vi "SetExit.vi"(6 "Legacy (f)?":bool, 8 "error in (no error)":errorcluster) -> (0 "error out":errorcluster)   [LabVIEW 2011]
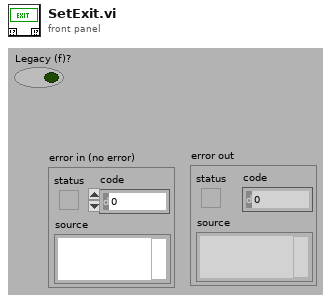
[diagram p1: front panel]
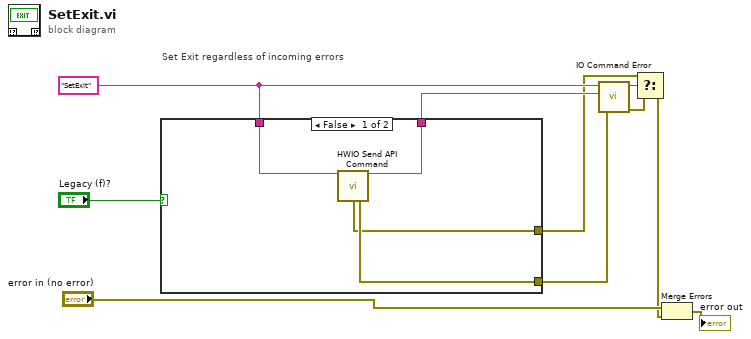
[diagram p0: block diagram]
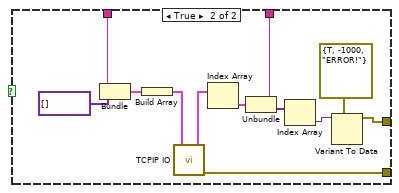
[diagram p2: hidden frame]
diagram:
  w10 = "SetExit"
  # "Set Exit regardless of incoming errors"
  n1 = case shown="False" "Legacy (f)?" {
    tunnel: w10 -> [w12 w24]
    tunnel: [w13 w22] -> w9
    tunnel: [w14 w16] -> w3
    tunnel: [w11 w15] -> w2
    frame False {
      n2 = call "HWIO Send API Command.vi"("Action"=w12) -> ("Action out"=w13:string, "HWError"=w11:errorcluster, "error out"=w14:errorcluster)  [unwired: 7 in, 5 out]
    }
    frame True {
      n3 = Bundle(w24, variant[] []) -> (w25:cluster{string, variant[]})  [unwired: 1 out]
      n4 = Build Array(w25) -> (w20:cluster{string, variant[]}[])
      n5 = call "TCPIP IO.vi"("Commands"=w20) -> ("error out"=w16:errorcluster, "Responses"=w21:cluster{string, variant[]}[])  [unwired: 2 in, 3 out]
      n6 = Index Array(array=w21) -> (element=w23:cluster{string, variant[]})  [unwired: 1 in]
      n7 = Unbundle(w23) -> (w22:string, w17:variant[])
      n8 = Index Array(array=w17) -> (element=w19:variant)  [unwired: 1 in]
      n9 = Variant To Data(type=errorcluster {"status"=TRUE, "code"=-1000, "source"="ERROR!"} ("error out"), Variant=w19) -> (data=w15:errorcluster)  [unwired: 1 in, 1 out]
    }
  }
  n10 = call "IO Command Error.vi"("error in (no error)"=w3, "Command Returned (\"\")"=w9, "Command Sent (\"\")"=w10) -> ("error out"=w4:errorcluster, "HW ERR?"=w5:bool)  [unwired: 3 out]
  n11 = Select(t=w2, s=w5, f=w4) -> (s? t:f=w6:errorcluster)
  n12 = Merge Errors("error in (no error)", w6) -> (→"error out":errorcluster)
